vi "Create Line of best fit equation.vi"(11 "Line to create equation for":cluster{"Points":cluster{"X":dbl, "Y":dbl}[]}) -> (1 "Y coefficient":dbl, 2 "X coefficient":dbl, 3 "Constant":dbl)   [LabVIEW 2016]
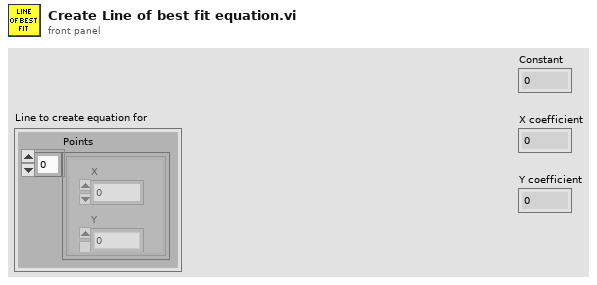
[diagram p1: front panel]
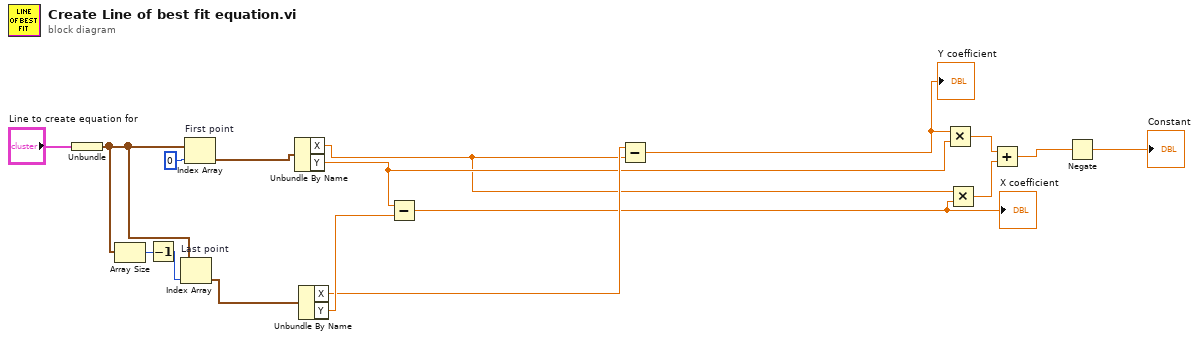
[diagram p0: block diagram]
diagram:
  n1 = Unbundle("Line to create equation for") -> ("Points"=w14:cluster{"X":dbl, "Y":dbl}[])
  n2 = Array Size(array=w14) -> (size(s)=w15:i32)
  n3 = Decrement(x=w15) -> (x-1=w13:i32)
  n4 = Index Array "Last point"(array=w14, index=w13) -> (element=w11:cluster{"X":dbl, "Y":dbl})
  n5 = Index Array "First point"(array=w14, index=0) -> (element=w12:cluster{"X":dbl, "Y":dbl})
  n6 = Unbundle By Name(w12) -> ("X"=w3:dbl, "Y"=w7:dbl)
  n7 = Unbundle By Name(w11) -> ("X"=w9:dbl, "Y"=w10:dbl)
  n8 = Subtract(x=w7, y=w10) -> (x-y=w2:dbl)
  "X coefficient" <- w2
  n9 = Subtract(x=w9, y=w3) -> (x-y=w8:dbl)
  "Y coefficient" <- w8
  n10 = Multiply(x=w8, y=w7) -> (x*y=w5:dbl)
  n11 = Multiply(x=w3, y=w2) -> (x*y=w6:dbl)
  n12 = Add(x=w5, y=w6) -> (x+y=w4:dbl)
  n13 = Negate(x=w4) -> (-x=→"Constant":dbl)
